vi "MulticolumnListbox - get selected.vi"(7 "Flights ref":refnum<vi>) -> (8 "ItemNames":string[][](array[string]))   [LabVIEW 2010, in "util.lvlib"]
uses:
  util.lvlib
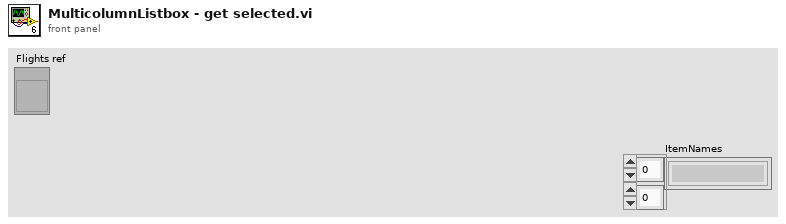
[diagram p1: front panel]
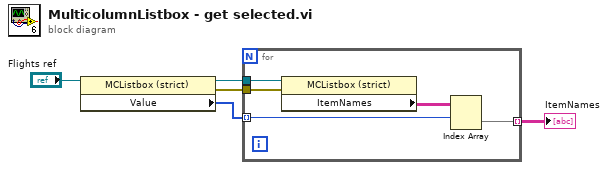
[diagram p0: block diagram]
diagram:
  n1 = property on="Eigenschaftsknoten" class="MCListbox (strict)"(reference="Flights ref") -> (reference out=w2:refnum<vi>, error out=w1:errorcluster, "Value"=w3:i32[])  [unwired: 1 in]
  n2 = for {
    tunnel: w3 -> [w10] mode=indexing
    tunnel: [w9] -> w5 mode=indexing
    tunnel: w2 -> [w8]
    tunnel: w1 -> [w7]
    n3 = property on="Eigenschaftsknoten" class="MCListbox (strict)"(reference=w8, error in=w7) -> ("ItemNames"=w6:string[][])  [unwired: 2 out]
    n4 = Index Array(array=w6, index (row)=w10) -> (element=w9:string[])  [unwired: 1 in]
  }
  "ItemNames" <- w5
